vi "Andor Format CrvNames.vi"(4 "WaveBands":T1(array[cluster]) {"WB End" min=1 max=255 step=1; "WB Start" min=1 max=255 step=1}, 6 "Noise Mode":T2=enum."Selected Curve", 7 "NoiseWindow":bool, 8 "error in (no err)":errorcluster, 10 "Accumulation":i32=1 min=1 max=256 step=1, 11 "numAreas":i32=1) -> (0 "error out":errorcluster, 1 "DatDisplayNm":string[](array[string]), 2 "VarParY":dbl[](array[numeric]), 3 "SubDatDisplayNm":string[](array[string]))   [LabVIEW 2019]
uses:
  <userlib>/ATSpectrograph/GUI/AndorNoiseCorr.ctl
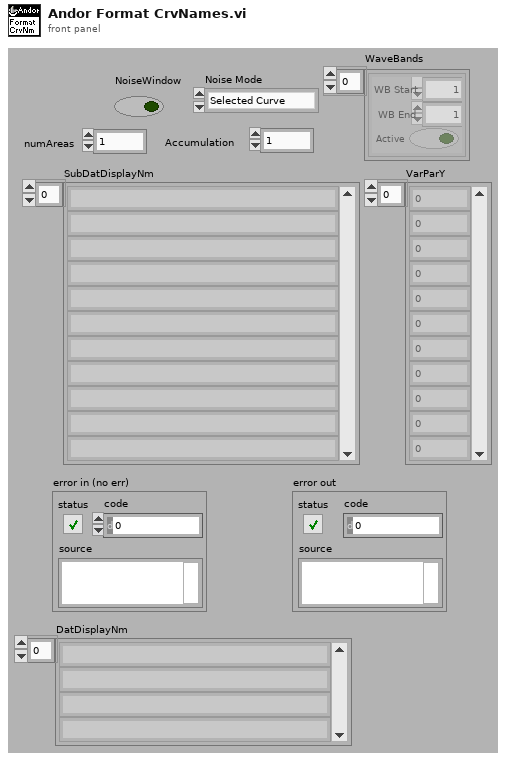
[diagram p1: front panel]
types:
  T1 = cluster{"WB Start":i32, "WB End":i32, "Active":bool}[]
  T2 = typedef "AndorNoiseCorr.ctl" = enum16{"Off", "Selected Curve", "One For Every Acq"}
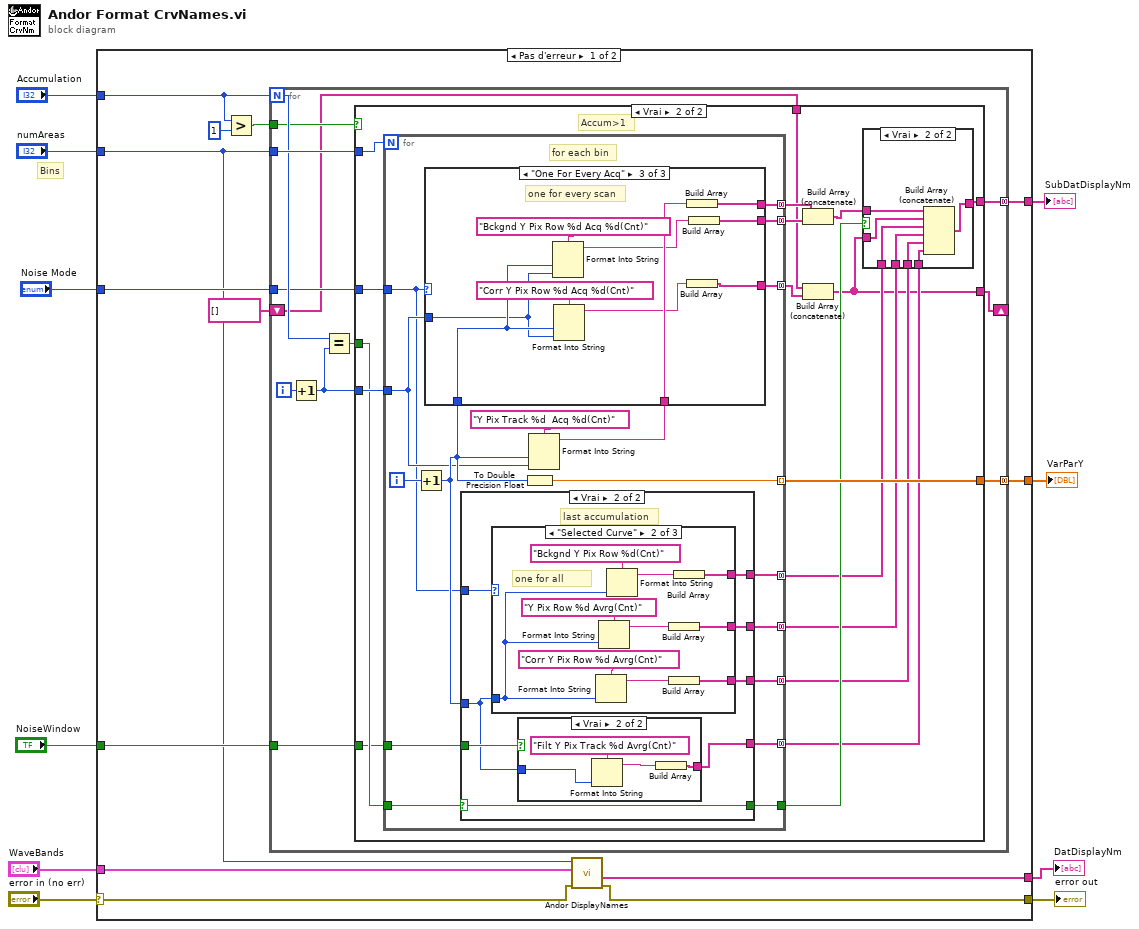
[diagram p0: block diagram]
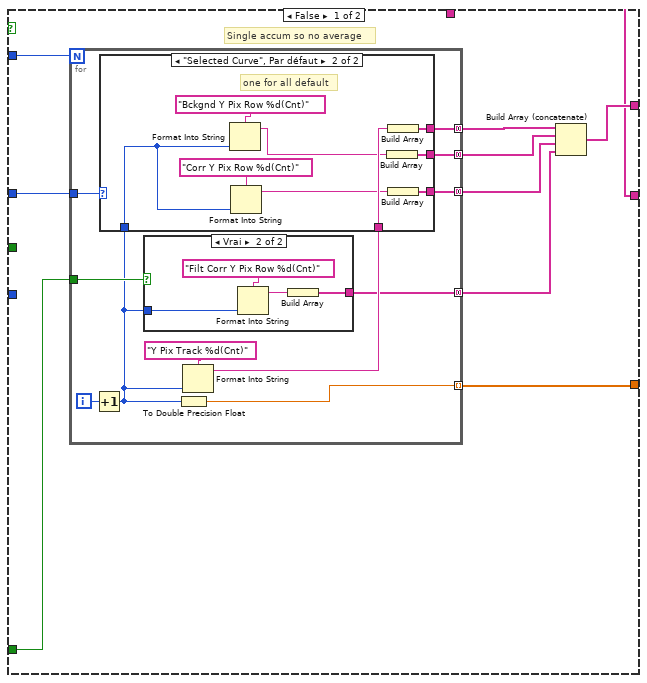
[diagram p2: hidden frame]
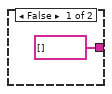
[diagram p3: hidden frame]
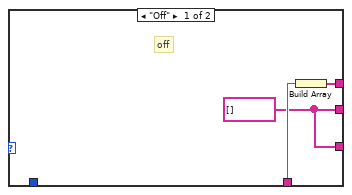
[diagram p4: hidden frame]
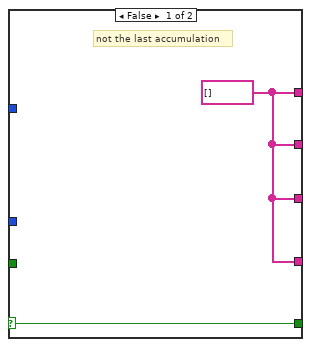
[diagram p6: hidden frame]
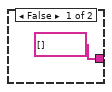
[diagram p7: hidden frame]
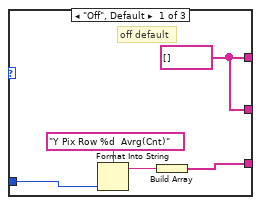
[diagram p8: hidden frame]
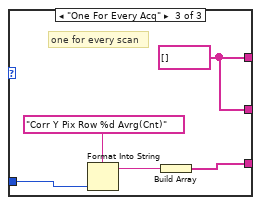
[diagram p9: hidden frame]
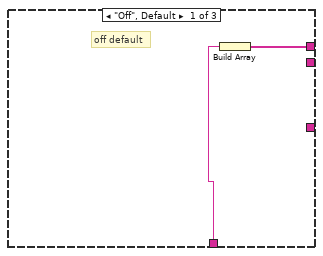
[diagram p10: hidden frame]
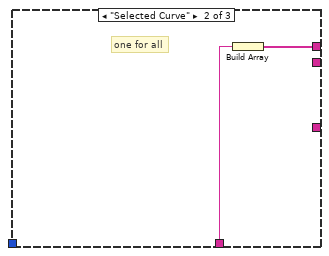
[diagram p11: hidden frame]
diagram:
  # "Bins"
  n1 = case shown="Pas d'erreur" "error in (no err)" {
    selector: "error in (no err)" -> [w12 w166]
    tunnel: "numAreas" -> [w14 _]
    tunnel: "Accumulation" -> [w21 _]
    tunnel: [w11 w166] -> w7
    tunnel: [w23 _] -> w6
    tunnel: [w22 _] -> w5
    tunnel: "NoiseWindow" -> [w18 _]
    tunnel: "Noise Mode" -> [w17 _]
    tunnel: [w13 _] -> w2
    tunnel: "WaveBands" -> [w15 _]
    frame No Error {
      n2 = Greater?(x=w21, y=1) -> (0:w19:bool)
      n3 = for {
        N: w21 -> [w30]
        tunnel: [w35] -> w23 mode=concatenating
        tunnel: [w34] -> w22 mode=concatenating
        tunnel: w14 -> [w33]
        tunnel: w19 -> [w26]
        tunnel: w18 -> [w28]
        tunnel: w17 -> [w27]
        shift-right: [w25] -> _
        shift-left: string[] [] -> [w24]
        i -> [w32]
        n4 = Increment(x=w32) -> (x+1=w31:i32)
        n5 = Equal?(x=w30, y=w31) -> (x = y?=w29:bool)
        n6 = case shown="Vrai" w26 {
          tunnel: [w40 w86] -> w35
          tunnel: [w44 w91] -> w34
          tunnel: w33 -> [w43 w90]
          tunnel: w31 -> [_ w89]
          tunnel: w29 -> [_ w88]
          tunnel: w28 -> [w42 w84]
          tunnel: w27 -> [w41 w83]
          tunnel: [w36 w74] -> w25
          tunnel: w24 -> [w36 w76]
          frame False {
            # "Single accum so no average"
            n7 = for {
              N: w43 -> [_]
              tunnel: [w56] -> w44 mode=indexing
              tunnel: [w52] -> w45 mode=concatenating
              tunnel: w42 -> [w48]
              tunnel: w41 -> [w51]
              tunnel: [w50] -> w39 mode=concatenating
              tunnel: [w49] -> w38 mode=concatenating
              tunnel: [w46] -> w37 mode=concatenating
              i -> [w55]
              n8 = Increment(x=w55) -> (x+1=w47:i32)
              n9 = case shown="Vrai" w48 {
                tunnel: w47 -> [_ w60]
                tunnel: [string[] [] w58] -> w46
                frame False {
                }
                frame True {
                  n10 = Format Into String(format string="Filt Corr Y Pix Row %d(Cnt)", w60) -> (resulting string=w59:string)  [unwired: 2 in, 1 out]
                  n11 = Build Array(w59) -> (w58:string[])
                }
              }
              n12 = To Double Precision Float(number=w47) -> (double precision float=w56:dbl)
              n13 = Format Into String(format string="Y Pix Track %d(Cnt)", w47) -> (resulting string=w53:string)  [unwired: 2 in, 1 out]
              n14 = case shown="\"Selected Curve\", Par défaut" w51 {
                tunnel: w53 -> [w64 w72]
                tunnel: [w63 w73] -> w52
                tunnel: w47 -> [_ w71]
                tunnel: [w62 w70] -> w50
                tunnel: [w62 w69] -> w49
                frame "Off" {
                  w62 = string[] []
                  # "off"
                  n15 = Build Array(w64) -> (w63:string[])
                }
                frame "Selected Curve", Default {
                  # "one for all default"
                  n16 = Format Into String(format string="Bckgnd Y Pix Row %d(Cnt)", w71) -> (resulting string=w65:string)  [unwired: 2 in, 1 out]
                  n17 = Format Into String(format string="Corr Y Pix Row %d(Cnt)", w71) -> (resulting string=w66:string)  [unwired: 2 in, 1 out]
                  n18 = Build Array(w65) -> (w69:string[])
                  n19 = Build Array(w72) -> (w73:string[])
                  n20 = Build Array(w66) -> (w70:string[])
                }
              }
            }
            n21 = Build Array (concatenate)(w45, w38, w39, w37) -> (w40:string[])
          }
          frame True {
            # "Accum>1"
            n22 = for {
              N: w90 -> [_]
              tunnel: [w116] -> w91 mode=indexing
              tunnel: [w113] -> w79 mode=concatenating
              tunnel: w89 -> [w107]
              tunnel: w88 -> [w111]
              tunnel: [w109] -> w85 mode=concatenating
              tunnel: [w108] -> w87
              tunnel: w84 -> [w105]
              tunnel: w83 -> [w106]
              tunnel: [w104] -> w80 mode=concatenating
              tunnel: [w103] -> w81 mode=concatenating
              tunnel: [w102] -> w82 mode=concatenating
              tunnel: [w101] -> w75 mode=concatenating
              tunnel: [w100] -> w78 mode=concatenating
              i -> [w112]
              # "for each bin"
              n23 = Increment(x=w112) -> (x+1=w110:i32)
              n24 = case shown="Vrai" w111 {
                selector: w111 -> [w118 w126]
                tunnel: w110 -> [_ w120]
                tunnel: [w117 w119] -> w109
                tunnel: [w118 w126] -> w108
                tunnel: w106 -> [_ w125]
                tunnel: w105 -> [_ w121]
                tunnel: [w117 w124] -> w104
                tunnel: [w117 w123] -> w103
                tunnel: [w117 w122] -> w102
                frame False {
                  w117 = string[] []
                  # "not the last accumulation"
                }
                frame True {
                  # "last accumulation"
                  n25 = case shown="\"Selected Curve\"" w125 {
                    tunnel: w120 -> [w134 w146 w151]
                    tunnel: [w132 w141 w149] -> w124
                    tunnel: [w132 w139 w149] -> w123
                    tunnel: [w133 w137 w147] -> w122
                    frame "Off", Default {
                      w132 = string[] []
                      # "off default"
                      n26 = Format Into String(format string="Y Pix Row %d  Avrg(Cnt)", w134) -> (resulting string=w136:string)  [unwired: 2 in, 1 out]
                      n27 = Build Array(w136) -> (w133:string[])
                    }
                    frame "Selected Curve" {
                      # "one for all"
                      n28 = Format Into String(format string="Corr Y Pix Row %d Avrg(Cnt)", w146) -> (resulting string=w138:string)  [unwired: 2 in, 1 out]
                      n29 = Format Into String(format string="Y Pix Row %d Avrg(Cnt)", w146) -> (resulting string=w140:string)  [unwired: 2 in, 1 out]
                      n30 = Format Into String(format string="Bckgnd Y Pix Row %d(Cnt)", w146) -> (resulting string=w142:string)  [unwired: 2 in, 1 out]
                      n31 = Build Array(w140) -> (w139:string[])
                      n32 = Build Array(w138) -> (w137:string[])
                      n33 = Build Array(w142) -> (w141:string[])
                    }
                    frame "One For Every Acq" {
                      w149 = string[] []
                      # "one for every scan"
                      n34 = Format Into String(format string="Corr Y Pix Row %d Avrg(Cnt)", w151) -> (resulting string=w150:string)  [unwired: 2 in, 1 out]
                      n35 = Build Array(w150) -> (w147:string[])
                    }
                  }
                  n36 = case shown="Vrai" w121 {
                    tunnel: w120 -> [_ w131]
                    tunnel: [string[] [] w130] -> w119
                    frame False {
                    }
                    frame True {
                      n37 = Format Into String(format string="Filt Y Pix Track %d Avrg(Cnt)", w131) -> (resulting string=w129:string)  [unwired: 2 in, 1 out]
                      n38 = Build Array(w129) -> (w130:string[])
                    }
                  }
                }
              }
              n39 = To Double Precision Float(number=w110) -> (double precision float=w116:dbl)
              n40 = Format Into String(format string="Y Pix Track %d  Acq %d(Cnt)", w110, w107) -> (resulting string=w114:string)  [unwired: 2 in, 1 out]
              n41 = case shown="\"One For Every Acq\"" w106 {
                tunnel: w114 -> [w153 w154 w165]
                tunnel: [w152 w155 w161] -> w113
                tunnel: w110 -> [_ _ w164]
                tunnel: w107 -> [_ _ w156]
                tunnel: [_ _ w163] -> w101
                tunnel: [_ _ w162] -> w100
                frame "Off", Default {
                  # "off default"
                  n42 = Build Array(w153) -> (w152:string[])
                }
                frame "Selected Curve" {
                  # "one for all"
                  n43 = Build Array(w154) -> (w155:string[])
                }
                frame "One For Every Acq" {
                  # "one for every scan"
                  n44 = Format Into String(format string="Bckgnd Y Pix Row %d Acq %d(Cnt)", w164, w156) -> (resulting string=w157:string)  [unwired: 2 in, 1 out]
                  n45 = Format Into String(format string="Corr Y Pix Row %d Acq %d(Cnt)", w164, w156) -> (resulting string=w158:string)  [unwired: 2 in, 1 out]
                  n46 = Build Array(w165) -> (w161:string[])
                  n47 = Build Array(w158) -> (w163:string[])
                  n48 = Build Array(w157) -> (w162:string[])
                }
              }
            }
            n49 = Build Array (concatenate)(w79, w78) -> (w77:string[])
            n50 = Build Array (concatenate)(w76, w75) -> (w74:string[])
            n51 = case shown="Vrai" w87 {
              tunnel: w77 -> [w92 w98]
              tunnel: [w92 w99] -> w86
              tunnel: w85 -> [_ w97]
              tunnel: w82 -> [_ w96]
              tunnel: w81 -> [_ w95]
              tunnel: w80 -> [_ w94]
              tunnel: w74 -> [_ w93]
              frame False {
              }
              frame True {
                n52 = Build Array (concatenate)(w98, w93, w94, w95, w96, w97) -> (w99:string[])
              }
            }
          }
        }
      }
      n53 = call <userlib>:"Andor DisplayNames.vi"("error in (no error)"=w12, "WaveBands"=w15, "numAreas"=w14) -> ("error out"=w11:errorcluster, "DatDisplayNm"=w13:string[])  [unwired: 7 in]
    }
    frame Error {
    }
  }
  "error out" <- w7
  "SubDatDisplayNm" <- w6
  "VarParY" <- w5
  "DatDisplayNm" <- w2
